vi "Get Error from DVR.vi"(8 "error in (no error)":errorcluster, 11 "Data Value Reference in":T1) -> (0 "error out":errorcluster, 2 "Error Out":errorcluster, 3 "Data Value Reference out":T1)   [LabVIEW 2011]
uses:
  Controls/DVR of CSV Tests Data.ctl
  Controls/CSVs Tests Data.ctl
  Controls/Test Column Data.ctl
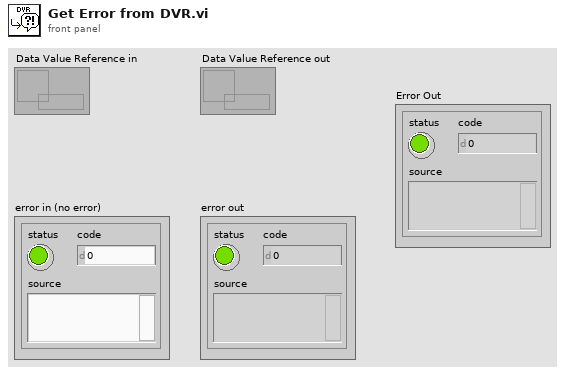
[diagram p1: front panel]
types:
  T1 = typedef "DVR of CSV Tests Data.ctl" = refnum<data-value>
  T2 = typedef "CSVs Tests Data.ctl" = cluster{"Test Data":T3[], "CsvPath":path, "LogPath":path, "Pass?":bool, "Error":errorcluster}
  T3 = typedef "Test Column Data.ctl" = cluster{"Chn":string, "ExpVals":dbl[], "TimeStamps":i64[], "NegTol":dbl, "PosTol":dbl}
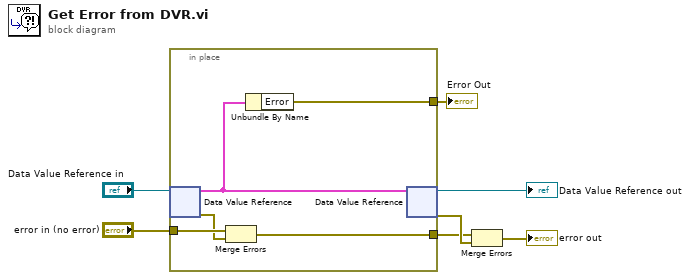
[diagram p0: block diagram]
diagram:
  n1 = in-place {
    in-place-border: "error in (no error)" -> [w12]
    in-place-border: [w9] -> w4
    in-place-border: [w8] -> w1
    n2 = in-place-dvr #1("Data Value Reference in") -> (w10:T2, w11:errorcluster)
    n3 = Merge Errors(w12, w11) -> (w9:errorcluster)
    n4 = Unbundle By Name(w10) -> ("Error"=w8:errorcluster)
    n5 = in-place-dvr #1(w10) -> (→"Data Value Reference out":T1, w5:errorcluster)
  }
  "Error Out" <- w1
  n6 = Merge Errors(w4, w5) -> (→"error out":errorcluster)
